vi "Robot Global Data.vi"() -> ()   [LabVIEW 2014]
doc: "This global VI can contain as many global variables as you need. Place a control on the panel, give it a good name. To read or write to it from a VI, drag the icon to the diagram of that VI. You can also drag from the project. Click on the node to change which global you access. You shouldn't have multiple locations writing to a global or it will cause a race-condition."
uses:
  <vilib>/Rock Robotics/WPI/Camera/WPI_CameraImageSize.ctl
  <vilib>/Rock Robotics/WPI/DriverStation/WPI_DriverStationRobotMode2.ctl
  Drivetrain Code/Drivetrain Control.ctl
  Drivetrain Code/Drivetrain Mode.ctl
  Common Code/Dashboard Control Data.ctl
  Common Code/Roller Control.ctl
  Common Code/Elevator DB Control.ctl
  Common Code/Elevator Presets.ctl
  Common Code/Encoder Control.ctl
  Common Code/Drivetrain Settings.ctl
  Pike/Pike DB Controls.ctl
  Common Code/commandCluster.ctl
  Common Code/IMU Data.ctl
  navX-MXP Library/COMMON/TypeDefs/Value TypeDefs/navX NAVX_CAL_STATUS.ctl
  navX-MXP Library/COMMON/TypeDefs/Value TypeDefs/navX NAVX_OP_STATUS.ctl
  Common Code/Vision Packet.ctl
  Dashboard Code/Vision/Vision Tote Data.ctl
  Common Code/Elevator Object Type.ctl
  Elevator/Elevator Control Command.ctl
  Elevator/Elevator Command.ctl
  Common Code/Elevator Mode.ctl
  Common Code/Elevator Idle Mode.ctl
  Common Code/Roller Indicators.ctl
  Common Code/Roller Mode Enum.ctl
  Common Code/Auto Roller Commands.ctl
  Common Code/Inner Roller States.ctl
  Sensors/Pot Data.ctl
  Rollers/Untip Can States.ctl
  Common Code/Elevator Status.ctl
  Common Code/Auto Elevator Indicators.ctl
  Common Code/Elevator State.ctl
  Rollers/Roller Modes.ctl
  Common Code/Roller Manual Bools.ctl
  Rollers/Really Real Manual Align.ctl
  Common Code/Encoder Values.ctl
  Common Code/Ultrasonic Indicators.ctl
  Common Code/Keyboard Packet.ctl
  Rollers/ThinRollerIndicators.ctl
  Common Code/Drivetrain Status.ctl
  Common Code/Dist Drive Status.ctl
  Common Code/Yaw Rate Compensation Indicators.ctl
  Autonomous/Auto DB settings.ctl
  Pike/Pike State.ctl
  Pike/Pike Mode.ctl
  Pike/Pike Command.ctl
  navX-MXP Library/navX-MXP IMU.lvlib
panel:
  out "Last State Auto":bool
  out "Pike Status":T3={"Motor Out"=0.0, "Current"=0.0, "Limit Switch"=FALSE, "Current Limit"=FALSE, "State"=enum."Going Up", "Command"=enum."Auto Up"}
  in  "Pike Command":T4
  in  "Reset IMU":bool
  in  "Recalibrate Gyro":bool
  in  "NavX Opened":bool
  in  "Can Grabber":bool
  in  "IMU Pitch Zero":dbl
  in  "IMU Roll Zero":dbl
  in  "IMU Yaw Zero":dbl
  out "Zero IMU":bool
  out "Gyro Calibration Complete":refnum<k4>
  in  "Auton Settings":T5
  out "Current Auto Command Data":T6
  out "Is IMU Reset?":bool
  out "Drivetrain Loop Time":i32
  out "100ms Loop Time":i32
  in  "Drivetrain Status":T7 {"Translation X" scale=-1.0..1.0; "X (Steer)" scale=-1.0..1.0; "Y (Throttle)" scale=-1.0..1.0}
  in  "Elevator IR override":bool
  in  "Keyboard Packet":T11
  out "Zeroing Rollers?":bool
  in  "Left Pot 0":dbl
  in  "Right Pot 0":dbl
  out "US Loop Time":i32
  out "Ultrasonic Data":T12
  out "Elevator Loop Time":i32
  out "Roller Loop Time":i32
  in  "Elevator Been Zeroed":bool
  out "Encoder Values":T14 {"Right Encoder"."Ticks" format="%#.6g"; "Center Encoder"."Ticks" format="%#.6g"; "Left Encoder"."Ticks" format="%#.6g"}
  in  "Roller Manual":T15
  in  "Roller Modes":T17={"Auto Roller Command"=enum."Grab Tote", "Roller Mode"=enum."Manual", "Override Intake Speed"=0.0}
  out "Automation Safe Mode?":bool
  out "Elevator Status Data":T20 {"Motor Out" scale=-1.0..1.0}
  out "Roller State Indicators":T24={"Rollers Closed?"=FALSE, "Roller Mode"=enum."Manual", "Auto Roller State"=enum."Grab Tote", "Tote Inside?"=FALSE, "Intake State"=enum."Acquire Tote", "Left Ping Dist"=0.0, "Right Ping Dist"=0.0, "Potentiometer Cluster"={"Left Pot Zero"=0.0, "Right Pot Zero"=0.0, "Left Potentiometer"=0.0, "Right Potentiometer"=0.0, "Left Pot Non Zero"=0.0, "Right Pot Non Zero"=0.0}, "PING Decision"=enum."Acquire Tote", "Left Arm Closed?"=FALSE, "Portrait?"=FALSE, "Right Arm Closed?"=FALSE, "Left Out"=0.0, "Right Out"=0.0, "Left Current"=0.0, "Right Current"=0.0, "Tote Load Complete?"=FALSE, "Untip Complete?"=FALSE, "Untip State"=enum."Idle", "Roller Safety Open"=FALSE} {"Right Out" scale=-1.0..1.0; "Left Out" scale=-1.0..1.0}
  in  "Elevator Command":T28={"Command"=enum."Idle", "Manual Motor Out"=0.0, "Manual Eject Piston"=FALSE, "Mode"=enum."Manual", "Override Limits"=FALSE, "Manual Stabilizer"=FALSE, "Manual Finger"=FALSE, "Store Trashcan?"=FALSE, "Hold Low?"=FALSE, "Idle Mode"=enum."Load Can", "HP Load"=FALSE, "Unstick"=FALSE, "Raw Height Set"=0.0, "Force Store"=FALSE}
  out "Gyro Value":dbl
  out "Vision Connected?":bool
  out "Vision Packet":T31
  out "IMU Data":T34 {"NAVX_OP_STATUS" items=["INITIALIZING", "SELFTEST_IN_PROGRESS", "ERROR", "IMU_AUTOCAL_IN_PROGRESS", "NORMAL"]; "NAVX_CAL_STATUS" items=["IMU_CAL_STATE_MASK"=3, "IMU_CAL_INPROGRESS"=0, "IMU_CAL_ACCUMULATE"=1, "IMU_CAL_COMPLETE"=2, "MAG_CAL_COMPLETE"=4, "BARO_CAL_COMPLETE"=8]}
  in  "IMU Gyro Zero X":dbl
  in  "IMU Gyro Zero Y":dbl
  in  "IMU Gyro Zero Z":dbl
  out "Auton Files Count":i32
  in  "Auton File Array":string[](array[string])
  in  "Selected Auton":string
  out "Auton File Index":i32
  in  "Auton File Names":string
  in  "Driver Station IP":u32
  in  "Dashboard Packet":T37={"Cam Exposure"=0.0, "Go to angle"=57.0, "Steer PID Gains"={"proportional gain (Kc)"=0.0624, "integral time (Ti, min)"=0.0, "derivative time (Td, min)"=0.002}, "Steer PID output Range"={"output high"=0.8, "output low"=-0.8}, "Pressure m \nValue"=34.774, "Pressure b \nValue"=-58.564, "Roller Command Cluster "={"Intake Speed"=1.0, "Turn In Speed"=0.8, "Unload Speed"=-1.0, "Turn Out Speed"=-0.8, "Ping Align Tolerance"=3.0, "Tote Range Threshold"=25.0, "Right Pot 0"=0.0, "Pot Threshold"=10.0, "Left Pot 0"=0.0, "Right Pot Scale"=100.0, "Left Pot Scale"=100.0, "Min Elevator Height"=12.0, "Eject Time"=1500.0, "Eject US Threshold"=10.0, "Anti-Twitch Time"=500, "Ping Caring Threshold"=15.0, "Pot Diff Threshold"=2.0, "Pinch Sustain"=500, "Absorb Give Up Threshold"=18.0, "Untip In Threshold"=20.0, "Untip Grab Range"=26.0, "Ultrasonic Hold Time"=500, "Landscape Absorb Time"=0, "Pot Use Wait Time"=250, "Can Turn Stop Range"=0.0, "HP Load Speed"=0.0, "Stick Multiplier"=0.0}, "Elevator"={"PID Output Range"={"output high"=1.0, "output low"=-1.0}, "PID gains"={"proportional gain (Kc)"=1.0, "integral time (Ti, min)"=0.0, "derivative time (Td, min)"=0.0}, "Height Tolerance"=0.25, " Encoder Constant"=0.003945, "Eject Time"=0.0, "Zeroing Speed"=1.0, "Presets"={"Pickup 2 w/ Tote"=27.0, "Pickup 2 w/ Trashcan"=40.0, "Pickup 3 w/ Tote"=40.0, "Pickup 3 w/ Trashcan"=46.0, "Bottom"=0.0, "Pickup 1 w/ Tote"=17.0, "Pickup Trashcan"=0.0, "Pickup 1 w/ Trashcan"=27.0, "Eject"=8.0, "Hold Low"=0.0, "Step add height"=7.0, "Untip Lift"=26.0, "Drop Stack"=1.0, "HP Load Hold"=32.0, "HP Load Drop"=10.0, "HP Load Hold Can"=0.0, "Store can max"=0.0, "HP Drag Score"=0.0, "HP Drag Finish"=0.0, "Finger trashcan avoid"=0.0, "Full"=0.0}, "Ping Detect Threshold"=3.0, "Trashcan Detect Threshold"=9.0, "Zero Filter Time"=30.0, "Stabilizer Open Time"=500.0, "Zero Creep Speed"=-0.2, "Max Current"=45.0, "Current Trip Time"=250.0, "Abort Pitch"=6.0, "Finger m"=0.0, "Finger b"=0.0, "Finger max "=0.0, "Finger Stabilizer"=0.0, "Finger Store"=0.0, "Finger Stop Store"=0.0, "Stabilizer Close Time"=0.0, "Finger min"=0.0, "Unstick gain"=0.0, "Full Detect Max"=0.0}, "Encoder Control"={"Left Tick Constant"=0.004057, "Right Tick Constant"=0.004057, "Center Tick Constant"=1.0, "Reset?"=FALSE, "Y Dist"={"PID gains"={"proportional gain (Kc)"=1.0, "integral time (Ti, min)"=0.0, "derivative time (Td, min)"=0.001}}, "X Dist"={"PID gains"={"proportional gain (Kc)"=0.0, "integral time (Ti, min)"=0.0, "derivative time (Td, min)"=0.0}}, "Y Stop Thresh"=0.25, "Y Stop Speed"=1.0, "X Stop Thresh"=0.25, "X Stop Speed"=1.0}, "Auton Settings"={"Drive Dist Window Size"=0.0}, "Drivetrain Settings"={"Gyro Tolerance"=2.0, "Strafe Correct max steer"=0.4, "Strafe Timer Wait"=250.0, "Throttle Ramp (ms)"=250.0, "Strafe Ramp (ms)"=250.0, "Angular rate compensation"=FALSE, "Throttle to Rate Scale"=0.0, "Rate compensation gain"=0.0, "Creep Steer"=0.0, "Creep Throttle"=0.0}, "Lance"={"Down Speed"=0.0, "Up Speed"=0.0, "Max Down Time"=0.0, "Max Up Time"=0.0, "Current Limit"=0.0}} {"Drivetrain Settings"."Rate compensation gain" format="%#_6f"; "Drivetrain Settings"."Throttle to Rate Scale" format="%#_6f"; "Encoder Control"."X Dist"."PID gains"."derivative time (Td, min)" format="%.3f"; "Encoder Control"."X Dist"."PID gains"."integral time (Ti, min)" format="%.3f"; "Encoder Control"."X Dist"."PID gains"."proportional gain (Kc)" format="%.3f"; "Encoder Control"."Y Dist"."PID gains"."derivative time (Td, min)" format="%.3f"; "Encoder Control"."Y Dist"."PID gains"."integral time (Ti, min)" format="%.3f"; "Encoder Control"."Y Dist"."PID gains"."proportional gain (Kc)" format="%.3f"; "Steer PID Gains"."derivative time (Td, min)" format="%.3f"; "Steer PID Gains"."integral time (Ti, min)" format="%.3f"; "Steer PID Gains"."proportional gain (Kc)" format="%.3f"}
  in  "Auton Command Array":T6[](array[typedef])
  in  "Drivetrain Command":T44={"Mode"=enum."Gyro Steer", "Steer"=0.0, "Y"=0.0, "Heading Target"=0.0, "Strafe X"=0.0, "Y Target"=0.0, "Strafe Target"=0.0, "X Max Speed"=0.0, "X Min Speed"=0.0, "Y Max Speed"=0.0, "Y Min Speed"=0.0, "Force strafe"=FALSE, "Pivot Speed"=0.0}
  in  "Robot Mode":T45
  in  "image size":T46=enum."320x240"
  in  "Enable Vision":bool
  out "Roller Indicators Thin":T47={"Rollers Closed?"=FALSE, "Roller Mode"=enum."Manual", "Left Out"=0.0, "Right Out"=0.0, "L Current"=1.0, "R Current"=1.0} {"Right Out" scale=-1.0..1.0; "Left Out" scale=-1.0..1.0}
  # "on = open"
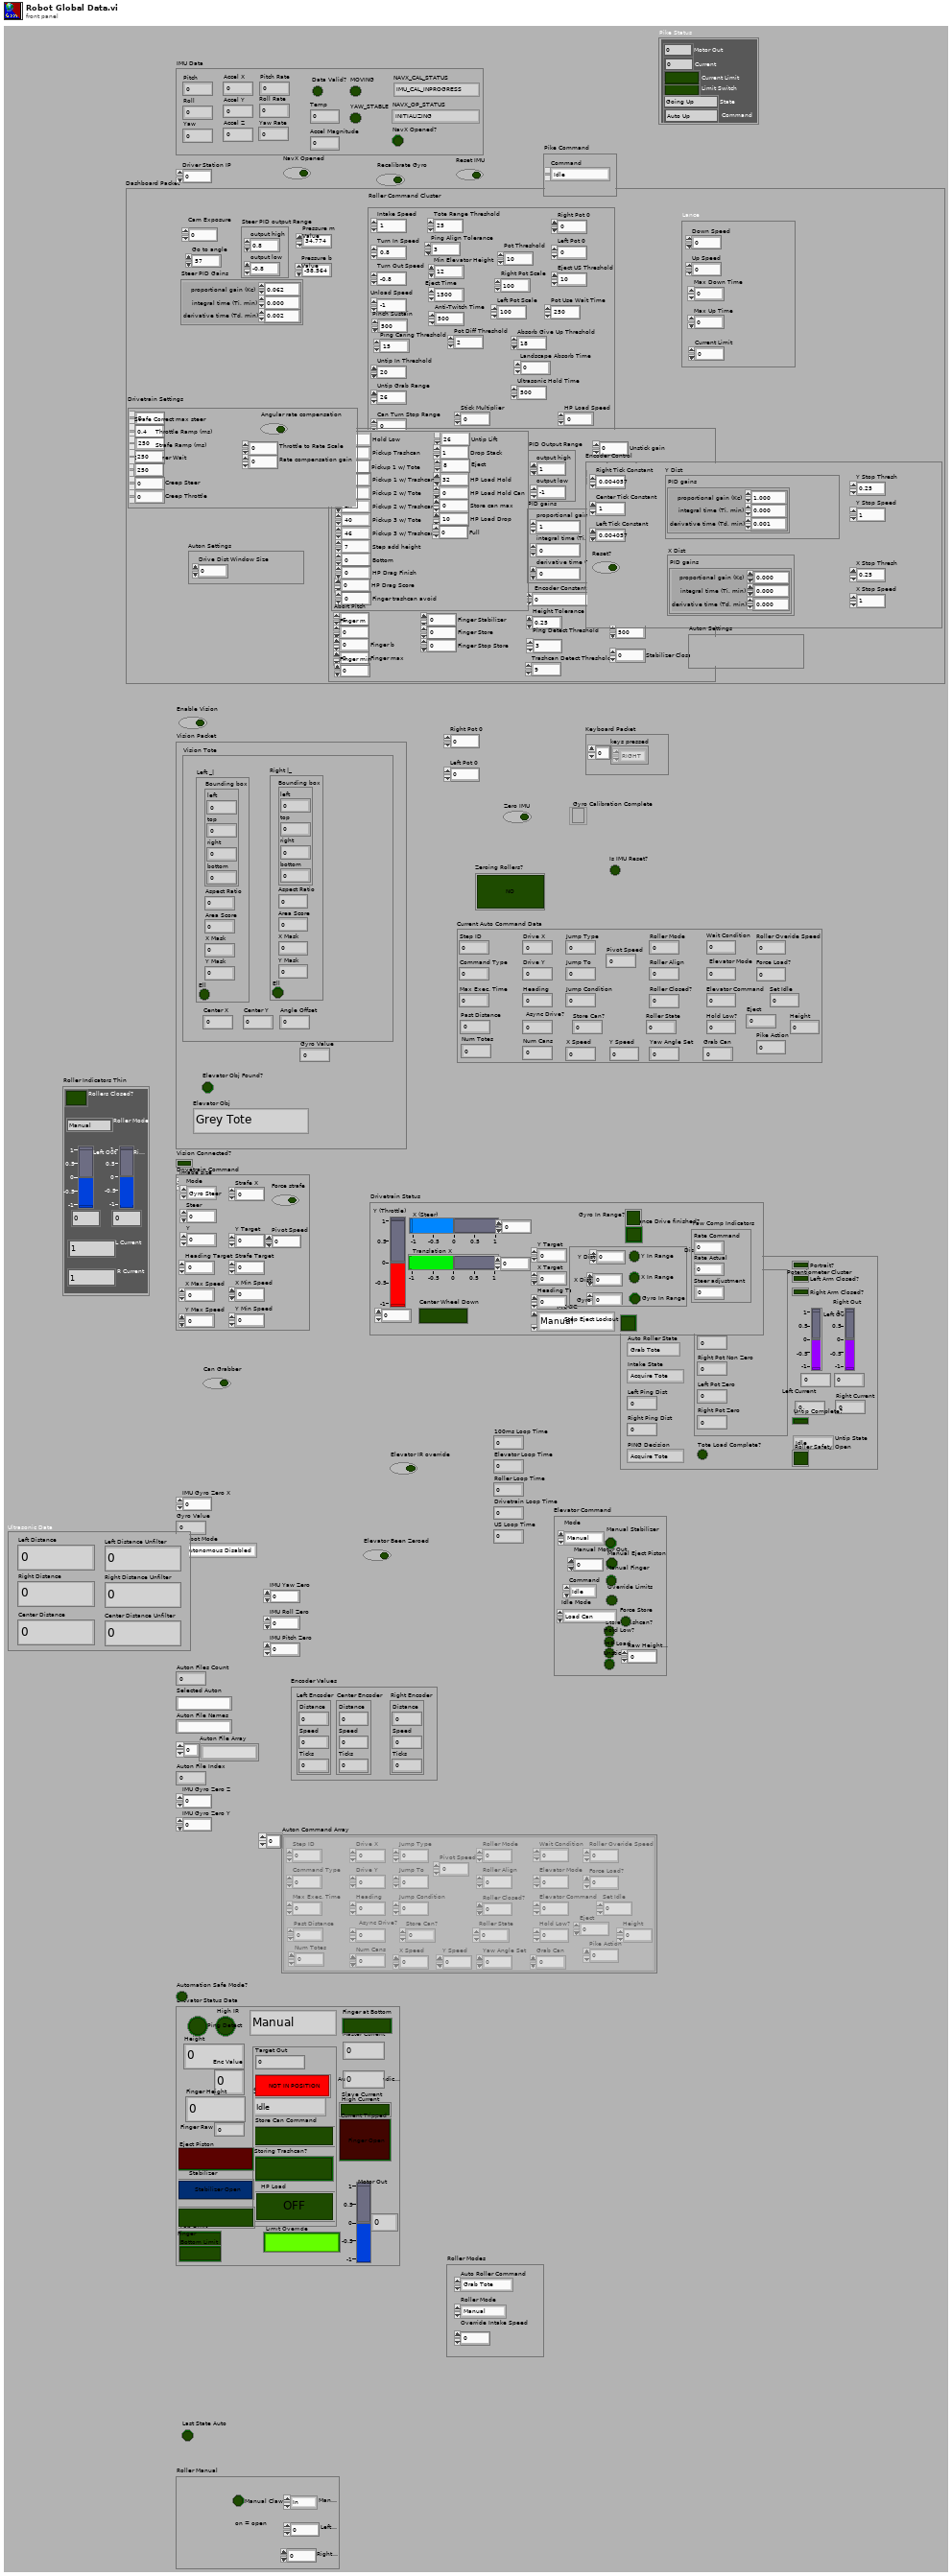
[diagram p1: front panel]
types:
  T1 = typedef "Pike State.ctl" = enum16{"Up", "Down", "Going Up", "Going Down"}
  T2 = typedef "Pike Mode.ctl" = enum16{"Idle", "Auto Down", "Auto Up", "Manual Down", "Manual Up"}
  T3 = cluster{"Motor Out":dbl, "Current":dbl, "Limit Switch":bool, "Current Limit":bool, "State":T1, "Command":T2}
  T4 = typedef "Pike Command.ctl" = cluster{"Command":T2}
  T5 = typedef "Auto DB settings.ctl" = cluster{}
  T6 = typedef "commandCluster.ctl" = cluster{"Step ID":i16, "Command Type":i16, "Drive X":sgl, "Drive Y":sgl, "Heading":sgl, "Max Exec. Time":i16, "Jump Type":i32, "Jump To":i16, "Jump Condition":i16, "Async Drive?":i16, "Roller Mode":i16, "Roller Align":i16, "Roller Closed?":i16, "Wait Condition":i16, "Elevator Mode":i16, "Elevator Command":i16, "Roller State":i16, "Hold Low?":i16, "Num Totes":i16, "Num Cans":dbl, "Past Distance":dbl, "Store Can?":dbl, "X Speed":dbl, "Y Speed":dbl, "Yaw Angle Set":dbl, "Grab Can":dbl, "Roller Overide Speed":dbl, "Force Load?":sgl, "Set Idle":sgl, "Eject":sgl, "Pike Action":sgl, "Pivot Speed":dbl, "Height":dbl}
  T7 = typedef "Drivetrain Status.ctl" = cluster{"Y (Throttle)":sgl, "X (Steer)":sgl, "Translation X":sgl, "Center Wheel Down":bool, "Mode":T8, "Distance Drive finished?":bool, "Y Target":sgl, "X Target":sgl, "Heading Target":sgl, "Dist Drive Status":T9, "Step Eject Lockout":bool, "Gyro In Range?":bool, "Yaw Comp Indicators":T10}
  T8 = typedef "Drivetrain Mode.ctl" = enum16{"Manual", "Gyro Steer", "Vision Steer", "Drive Distance", "Yaw Rate Compensate"}
  T9 = typedef "Dist Drive Status.ctl" = cluster{"Y In Range":bool, "X In Range":bool, "Gyro In Range":bool, "Y Dist":dbl, "X Dist":dbl, "Gyro":dbl}
  T10 = typedef "Yaw Rate Compensation Indicators.ctl" = cluster{"Rate Command":sgl, "Rate Actual":sgl, "Steer adjustment":sgl}
  T11 = typedef "Keyboard Packet.ctl" = cluster{"keys pressed":enum16{"0", "1", "2", "3", "4", "5", "6", "7", "8", "9", "A", "B", "C", "D", "E", "F", "G", "H", "I", "J", "K", "L", "M", "N", "O", "P", "Q", "R", "S", "T", "U", "V", "W", "X", "Y", "Z", "F1", "F2", "F3", "F4", "F5", "F6", "F7", "F8", "F9", "F10", "F11", "F12", "F13", "F14", "F15", "ADD", "BACK", "BACKSLASH", "CAPITAL", "COMMA", "DECIMAL", "DELETE", "DIVIDE", "DOWN", "END", "EQUALS", "ESCAPE", "GRAVE (`)", "HOME", "INSERT", "LBRACKET", "LCONTROL", "LEFT", "L ALT", "LSHIFT", "LWIN", "MINUS", "MULTIPLY", "NEXT", "NUMLOCK", "NUMPAD_0", "NUMPAD_1", "NUMPAD_2", "NUMPAD_3", "NUMPAD_4", "NUMPAD_5", "NUMPAD_6", "NUMPAD_7", "NUMPAD_8", "NUMPAD_9", "PAUSE", "PERIOD", "PRIOR (PG UP)", "RBRACKET", "RCONTROL", "RETURN", "RIGHT", "R ALT", "RSHIFT", "RWIN", "SCROLL", "SEMICOLON", "SLASH", "SPACE", "SUBTRACT", "TAB", "UP", "ENTER (num pad)", "' (quote)"}[]}
  T12 = typedef "Ultrasonic Indicators.ctl" = cluster{"Left Distance":dbl, "Right Distance":dbl, "Center Distance":dbl, "Left Distance Unfilter":dbl, "Right Distance Unfilter":dbl, "Center Distance Unfilter":dbl}
  T13 = typedef "Encoder Values.ctl" = cluster{"Distance":dbl, "Speed":dbl, "Ticks":dbl}
  T14 = cluster{"Left Encoder":T13, "Center Encoder":T13, "Right Encoder":T13}
  T15 = typedef "Roller Manual Bools.ctl" = cluster{"Manual Claw":bool, "Manual Align":T16, "Left Speed":dbl, "Right Speed":dbl}
  T16 = typedef "Really Real Manual Align.ctl" = enum16{"In", "Left", "Right", "Out", "Idle", "HP Load", "Speeds"}
  T17 = typedef "Roller Modes.ctl" = cluster{"Auto Roller Command":T18, "Roller Mode":T19, "Override Intake Speed":dbl}
  T18 = typedef "Auto Roller Commands.ctl" = enum16{"Drag Tote", "Grab Tote", "Idle", "Eject Tote", "Untip Can", "Grab Can"}
  T19 = typedef "Roller Mode Enum.ctl" = enum16{"Manual", "Safe", "Auto"}
  T20 = typedef "Elevator Status.ctl" = cluster{"Height":dbl, "Enc Value":dbl, "Limit Override":bool, "Mode":T21, "High IR":bool, "Motor Out":dbl, "Ping Detect":bool, "Auto Elevator Indicators":T22, "Master Current":dbl, "Slave Current":dbl, "High Current":bool, "Current Tripped":bool, "Top Limit":bool, "Bottom Limit":bool, "Eject Piston":bool, "Stabilizer":bool, "Finger":bool, "Finger Height":dbl, "Finger Raw":dbl, "Finger at Bottom":bool}
  T21 = typedef "Elevator Mode.ctl" = enum16{"Manual", "Safe", "Auto"}
  T22 = typedef "Auto Elevator Indicators.ctl" = cluster{"Target Out":dbl, "Storing Trashcan?":bool, "State":T23, "In Range":bool, "Store Can Command":bool, "HP Load":bool}
  T23 = typedef "Elevator State.ctl" = enum16{"Idle", "Goto Load Position", "Wait for Load", "Load Drop", "Load Lift", "Drop Stack", "Goto Eject Position", "Eject ", "Raise Trashcan", "Open Stabilizer", "Untip Drop", "Untip Wait", "Untip Lift", "Abort Load", "HP Load Wait", "HP Load Drop", "HP Load Lift", "HP Load Abort", "Close Stabilizer", "HP Load Unfinish", "HP Load Score", "HP Load Finish", "HP Goto Finish Down", "HP Goto Finish Up", "Full"}
  T24 = typedef "Roller Indicators.ctl" = cluster{"Rollers Closed?":bool, "Roller Mode":T19, "Auto Roller State":T18, "Tote Inside?":bool, "Intake State":T25, "Left Ping Dist":sgl, "Right Ping Dist":sgl, "Potentiometer Cluster":T26, "PING Decision":T25, "Left Arm Closed?":bool, "Portrait?":bool, "Right Arm Closed?":bool, "Left Out":sgl, "Right Out":sgl, "Left Current":sgl, "Right Current":sgl, "Tote Load Complete?":bool, "Untip Complete?":bool, "Untip State":T27, "Roller Safety Open":bool}
  T25 = typedef "Inner Roller States.ctl" = enum16{"Turn Tote Portrait", "Acquire Tote", "Absorb Tote", "Turn Tote Right", "Turn Tote Left", "Acquire Can", "Absorb Can", "Turn Can", "Hold Tote"}
  T26 = typedef "Pot Data.ctl" = cluster{"Left Pot Zero":sgl, "Right Pot Zero":sgl, "Left Potentiometer":sgl, "Right Potentiometer":sgl, "Left Pot Non Zero":sgl, "Right Pot Non Zero":sgl}
  T27 = typedef "Untip Can States.ctl" = enum16{"Release Can", "Catch Can", "Idle"}
  T28 = typedef "Elevator Control Command.ctl" = cluster{"Command":T29, "Manual Motor Out":dbl, "Manual Eject Piston":bool, "Mode":T21, "Override Limits":bool, "Manual Stabilizer":bool, "Manual Finger":bool, "Store Trashcan?":bool, "Hold Low?":bool, "Idle Mode":T30, "HP Load":bool, "Unstick":bool, "Raw Height Set":dbl, "Force Store":bool}
  T29 = typedef "Elevator Command.ctl" = enum16{"Idle", "Load 1", "Load 2", "Load 3", "Drop Stack", "Eject Stack", "Untip Trashcan", "Load Trashcan", "HP Load", "HP Score"}
  T30 = typedef "Elevator Idle Mode.ctl" = enum16{"Load 1", "Load 2", "Load 3", "Load Can", "Untip Can", "Step Load", "Drop Stack", "Raw Height"}
  T31 = typedef "Vision Packet.ctl" = cluster{"Vision Tote":T32, "Gyro Value":dbl, "Elevator Obj Found?":bool, "Elevator Obj":T33}
  T32 = typedef "Vision Tote Data.ctl" = cluster{"Left _|":cluster{"Bounding box":cluster{"left":dbl, "top":dbl, "right":dbl, "bottom":dbl}, "Aspect Ratio":dbl, "Area Score":dbl, "X Mask":dbl, "Y Mask":dbl, "Ell":bool}, "Right |_":cluster{"Bounding box":cluster{"left":dbl, "top":dbl, "right":dbl, "bottom":dbl}, "Aspect Ratio":dbl, "Area Score":dbl, "X Mask":dbl, "Y Mask":dbl, "Ell":bool}, "Center X":dbl, "Center Y":dbl, "Angle Offset":dbl}
  T33 = typedef "Elevator Object Type.ctl" = enum16{"Grey Tote", "Yellow Tote", "Trash Can"}
  T34 = typedef "IMU Data.ctl" = cluster{"Pitch":sgl, "Roll":sgl, "Yaw":sgl, "Data Valid?":bool, "Temp":sgl, "MOVING":bool, "NAVX_CAL_STATUS":T35, "NAVX_OP_STATUS":T36, "YAW_STABLE":bool, "Accel X":sgl, "Accel Y":sgl, "Accel Z":sgl, "Accel Magnitude":sgl, "Pitch Rate":sgl, "Roll Rate":sgl, "Yaw Rate":sgl, "NavX Opened?":bool}
  T35 = typedef "navX-MXP IMU.lvlib/navX NAVX_CAL_STATUS.ctl" = u8
  T36 = typedef "navX-MXP IMU.lvlib/navX NAVX_OP_STATUS.ctl" = u8
  T37 = typedef "Dashboard Control Data.ctl" = cluster{"Cam Exposure":dbl, "Go to angle":dbl, "Steer PID Gains":cluster{"proportional gain (Kc)":dbl, "integral time (Ti, min)":dbl, "derivative time (Td, min)":dbl}, "Steer PID output Range":cluster{"output high":dbl, "output low":dbl}, "Pressure m \nValue":dbl, "Pressure b \nValue":dbl, "Roller Command Cluster ":T38, "Elevator":T39, "Encoder Control":T41, "Auton Settings":cluster{"Drive Dist Window Size":dbl}, "Drivetrain Settings":T42, "Lance":T43}
  T38 = typedef "Roller Control.ctl" = cluster{"Intake Speed":dbl, "Turn In Speed":dbl, "Unload Speed":dbl, "Turn Out Speed":dbl, "Ping Align Tolerance":dbl, "Tote Range Threshold":dbl, "Right Pot 0":dbl, "Pot Threshold":dbl, "Left Pot 0":dbl, "Right Pot Scale":dbl, "Left Pot Scale":dbl, "Min Elevator Height":dbl, "Eject Time":dbl, "Eject US Threshold":dbl, "Anti-Twitch Time":u32, "Ping Caring Threshold":dbl, "Pot Diff Threshold":dbl, "Pinch Sustain":u32, "Absorb Give Up Threshold":dbl, "Untip In Threshold":dbl, "Untip Grab Range":dbl, "Ultrasonic Hold Time":u32, "Landscape Absorb Time":u32, "Pot Use Wait Time":u32, "Can Turn Stop Range":dbl, "HP Load Speed":dbl, "Stick Multiplier":dbl}
  T39 = typedef "Elevator DB Control.ctl" = cluster{"PID Output Range":cluster{"output high":dbl, "output low":dbl}, "PID gains":cluster{"proportional gain (Kc)":dbl, "integral time (Ti, min)":dbl, "derivative time (Td, min)":dbl}, "Height Tolerance":sgl, " Encoder Constant":dbl, "Eject Time":sgl, "Zeroing Speed":sgl, "Presets":T40, "Ping Detect Threshold":sgl, "Trashcan Detect Threshold":sgl, "Zero Filter Time":dbl, "Stabilizer Open Time":dbl, "Zero Creep Speed":dbl, "Max Current":dbl, "Current Trip Time":dbl, "Abort Pitch":dbl, "Finger m":dbl, "Finger b":dbl, "Finger max ":dbl, "Finger Stabilizer":dbl, "Finger Store":dbl, "Finger Stop Store":dbl, "Stabilizer Close Time":dbl, "Finger min":dbl, "Unstick gain":dbl, "Full Detect Max":dbl}
  T40 = typedef "Elevator Presets.ctl" = cluster{"Pickup 2 w/ Tote":sgl, "Pickup 2 w/ Trashcan":sgl, "Pickup 3 w/ Tote":sgl, "Pickup 3 w/ Trashcan":sgl, "Bottom":sgl, "Pickup 1 w/ Tote":sgl, "Pickup Trashcan":sgl, "Pickup 1 w/ Trashcan":sgl, "Eject":sgl, "Hold Low":sgl, "Step add height":sgl, "Untip Lift":dbl, "Drop Stack":dbl, "HP Load Hold":dbl, "HP Load Drop":dbl, "HP Load Hold Can":dbl, "Store can max":dbl, "HP Drag Score":dbl, "HP Drag Finish":dbl, "Finger trashcan avoid":dbl, "Full":dbl}
  T41 = typedef "Encoder Control.ctl" = cluster{"Left Tick Constant":dbl, "Right Tick Constant":dbl, "Center Tick Constant":dbl, "Reset?":bool, "Y Dist":cluster{"PID gains":cluster{"proportional gain (Kc)":dbl, "integral time (Ti, min)":dbl, "derivative time (Td, min)":dbl}}, "X Dist":cluster{"PID gains":cluster{"proportional gain (Kc)":dbl, "integral time (Ti, min)":dbl, "derivative time (Td, min)":dbl}}, "Y Stop Thresh":dbl, "Y Stop Speed":dbl, "X Stop Thresh":dbl, "X Stop Speed":dbl}
  T42 = typedef "Drivetrain Settings.ctl" = cluster{"Gyro Tolerance":sgl, "Strafe Correct max steer":sgl, "Strafe Timer Wait":sgl, "Throttle Ramp (ms)":sgl, "Strafe Ramp (ms)":sgl, "Angular rate compensation":bool, "Throttle to Rate Scale":sgl, "Rate compensation gain":sgl, "Creep Steer":sgl, "Creep Throttle":sgl}
  T43 = typedef "Pike DB Controls.ctl" = cluster{"Down Speed":dbl, "Up Speed":dbl, "Max Down Time":dbl, "Max Up Time":dbl, "Current Limit":dbl}
  T44 = typedef "Drivetrain Control.ctl" = cluster{"Mode":T8, "Steer":dbl, "Y":dbl, "Heading Target":dbl, "Strafe X":dbl, "Y Target":dbl, "Strafe Target":dbl, "X Max Speed":dbl, "X Min Speed":dbl, "Y Max Speed":dbl, "Y Min Speed":dbl, "Force strafe":bool, "Pivot Speed":dbl}
  T45 = typedef "WPI_DriverStationRobotMode2.ctl" = enum16{"Autonomous Disabled", "Autonomous Enabled", "Teleop Disabled", "Teleop Enabled", "Disconnected", "Finish", "Test Disabled", "Test Enabled", "Emergency Stopped"}
  T46 = typedef "WPI_CameraImageSize.ctl" = enum16{"640x480", "320x240", "160x120", "Custom"}
  T47 = typedef "ThinRollerIndicators.ctl" = cluster{"Rollers Closed?":bool, "Roller Mode":T19, "Left Out":dbl, "Right Out":dbl, "L Current":dbl, "R Current":dbl}
diagram:
